vi "Ex4.vi"() -> ()   [LabVIEW 2012]
doc: "Example VI: reads in and writes to Baxter's joint states"
uses:
  <userlib>/ROS for LabVIEW Software/ROS/Code/JointPositions.ctl
  <userlib>/ROS for LabVIEW Software/ROS/Code/Slider.ctl
panel:
  in  "Bring Arms In":bool
  in  "Reset to Zero":bool
  in  "Joint Positions":T1 {"left_w2" scale=-180.0..180.0; "left_w1" scale=-180.0..180.0; "left_w0" scale=-180.0..180.0; "left_e1" scale=-180.0..180.0; "left_e0" scale=-180.0..180.0; "left_s1" scale=-180.0..180.0; "left_s0" scale=-180.0..180.0; "right_s1" scale=-180.0..180.0; "right_s0" scale=-180.0..180.0; "right_w2" scale=-180.0..180.0; "right_e1" scale=-180.0..180.0; "right_e0" scale=-180.0..180.0; "right_w0" scale=-180.0..180.0; "right_w1" scale=-180.0..180.0}
  in  "stop":bool
  # "Control Baxter's Arms using the supplied Position Controller"
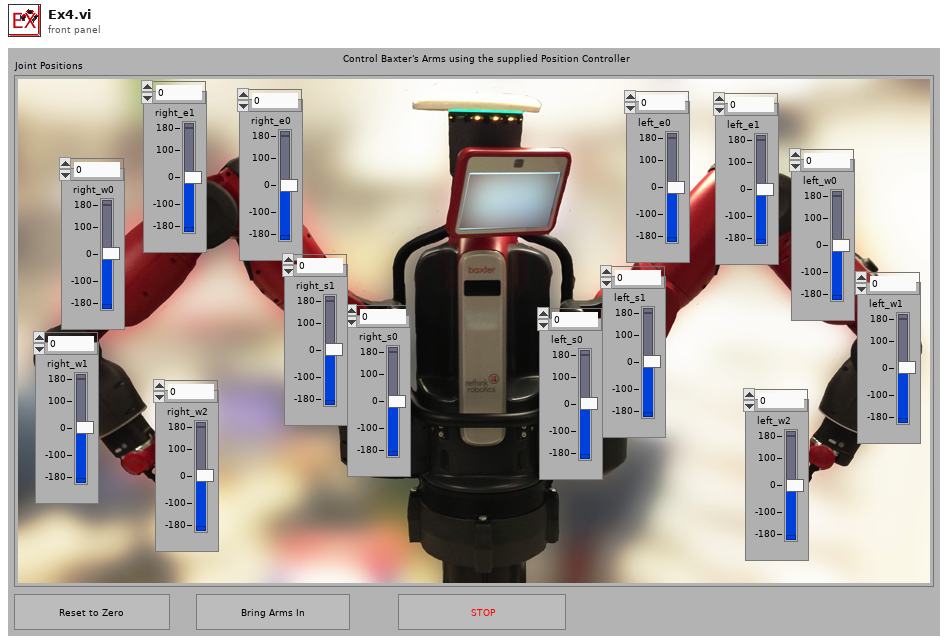
[diagram p1: front panel]
types:
  T1 = typedef "JointPositions.ctl" = cluster{"left_e0":T2, "left_e1":T2, "left_s0":T2, "left_s1":T2, "left_w0":T2, "left_w1":T2, "left_w2":T2, "right_e0":T2, "right_e1":T2, "right_s0":T2, "right_s1":T2, "right_w0":T2, "right_w1":T2, "right_w2":T2}
  T2 = typedef "Slider.ctl" = dbl
  T3 = cluster{"Joint Name":string, "Position":dbl, "Velocity":dbl, "Effort":dbl}[]
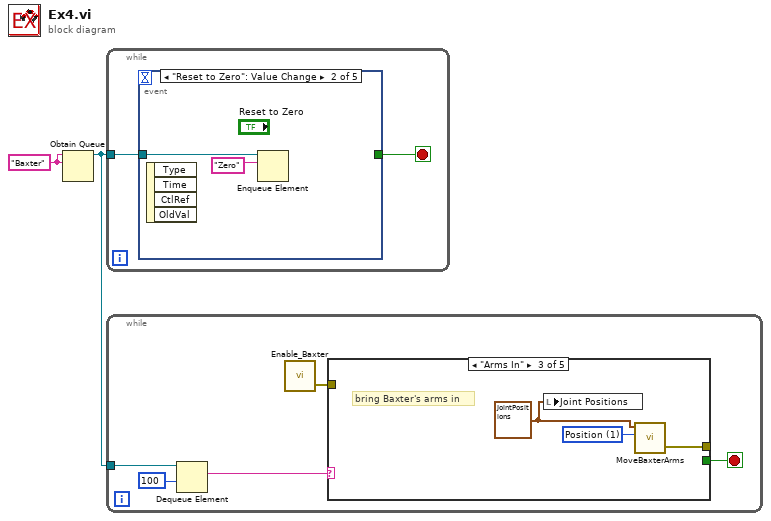
[diagram p0: block diagram]
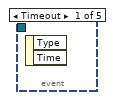
[diagram p2: hidden frame]
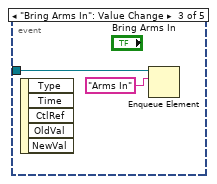
[diagram p3: hidden frame]
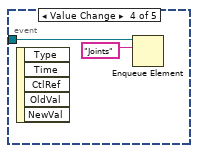
[diagram p4: hidden frame]
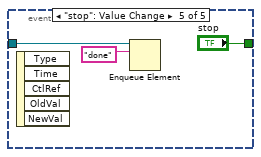
[diagram p5: hidden frame]
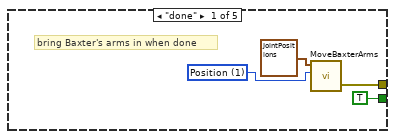
[diagram p6: hidden frame]
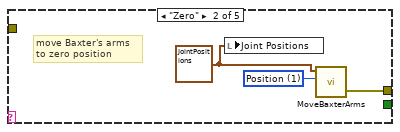
[diagram p7: hidden frame]
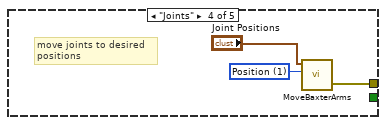
[diagram p8: hidden frame]
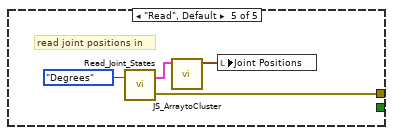
[diagram p9: hidden frame]
diagram:
  w1 = "Baxter" ("name (unnamed)")
  n1 = Obtain Queue(name (unnamed)=w1, element data type=w1) -> (queue out=w2:refnum<queue>)  [unwired: 3 in, 2 out]
  n2 = while {
    tunnel: w2 -> [w3]
    stop <- w4 stop-if-true
    n3 = event shown="[1] \"Reset to Zero\": Value Change" {
      selector: _ -> [_ _ _ _ _]
      dyn-events: _ -> [_ _ _ _ _]
      timeout: _ -> [_ _ _ _ _]
      tunnel: [_ _ _ _ "stop"] -> w4
      tunnel: w3 -> [_ w5 w7 w9 w12]
      event Timeout {
        n4 = event-data() -> ()  [unwired: 1 in, 2 out]
      }
      event "Reset to Zero": Value Change {
        n5 = event-data() -> ()  [unwired: 1 in, 4 out]
        n6 = Enqueue Element(queue=w5, element="Zero") -> ()  [unwired: 2 in, 3 out]
      }
      event "Bring Arms In": Value Change {
        n7 = event-data() -> ()  [unwired: 1 in, 5 out]
        n8 = Enqueue Element(queue=w7, element="Arms In") -> ()  [unwired: 2 in, 3 out]
      }
      event Value Change {
        n9 = event-data() -> ()  [unwired: 1 in, 5 out]
        n10 = Enqueue Element(queue=w9, element="Joints") -> ()  [unwired: 2 in, 3 out]
      }
      event "stop": Value Change {
        n11 = event-data() -> ()  [unwired: 1 in, 5 out]
        n12 = Enqueue Element(queue=w12, element="done") -> ()  [unwired: 2 in, 3 out]
      }
    }
  }
  n13 = while {
    tunnel: w2 -> [w18]
    stop <- w16 stop-if-true
    n14 = Dequeue Element(queue=w18, timeout in ms (-1)=100) -> (element=w17:string)  [unwired: 1 in, 3 out]
    n15 = call <userlib>:"Enable_Baxter.vi"() -> ("error out"=w14:errorcluster)  [unwired: 4 in]
    n16 = case shown="\"Arms In\"" w17 {
      tunnel: [TRUE ("stop") _ _ _ _] -> w16
      tunnel: [w19 w23 w26 w29 w32] -> _
      tunnel: w14 -> [_ _ _ _ _]
      frame "done" {
        w21 = u8 1 items=["Position"=1, "Velocity"=2, "Effort"=3] ("Mode")
        # "bring Baxter's arms in when done"
        n17 = call <userlib>:"MoveBaxterArms.vi"("Parameters"=T1 {"left_e0"=0.0, "left_e1"=90.0, "left_s0"=-30.0, "left_s1"=0.0, "left_w0"=0.0, "left_w1"=0.0, "left_w2"=0.0, "right_e0"=0.0, "right_e1"=90.0, "right_s0"=30.0, "right_s1"=0.0, "right_w0"=0.0, "right_w1"=0.0, "right_w2"=0.0} ("Joint Positions 2"), "Mode"=w21) -> ("error out"=w19:errorcluster)  [unwired: 4 in]
      }
      frame "Zero" {
        w24 = u8 1 items=["Position"=1, "Velocity"=2, "Effort"=3] ("Mode")
        w25 = T1 {"left_e0"=0.0, "left_e1"=0.0, "left_s0"=0.0, "left_s1"=0.0, "left_w0"=0.0, "left_w1"=0.0, "left_w2"=0.0, "right_e0"=0.0, "right_e1"=0.0, "right_s0"=0.0, "right_s1"=0.0, "right_w0"=0.0, "right_w1"=0.0, "right_w2"=0.0} ("Joint Positions 2")
        # "move Baxter's arms\nto zero position"
        n18 = local write "Joint Positions"(w25) -> ()
        n19 = call <userlib>:"MoveBaxterArms.vi"("Parameters"=w25, "Mode"=w24) -> ("error out"=w23:errorcluster)  [unwired: 4 in]
      }
      frame "Arms In" {
        w27 = u8 1 items=["Position"=1, "Velocity"=2, "Effort"=3] ("Mode")
        w28 = T1 {"left_e0"=0.0, "left_e1"=90.0, "left_s0"=-30.0, "left_s1"=0.0, "left_w0"=0.0, "left_w1"=0.0, "left_w2"=0.0, "right_e0"=0.0, "right_e1"=90.0, "right_s0"=30.0, "right_s1"=0.0, "right_w0"=0.0, "right_w1"=0.0, "right_w2"=0.0} ("Joint Positions 2")
        # "bring Baxter's arms in"
        n20 = local write "Joint Positions"(w28) -> ()
        n21 = call <userlib>:"MoveBaxterArms.vi"("Parameters"=w28, "Mode"=w27) -> ("error out"=w26:errorcluster)  [unwired: 4 in]
      }
      frame "Joints" {
        w30 = u8 1 items=["Position"=1, "Velocity"=2, "Effort"=3] ("Mode")
        # "move joints to desired\npositions"
        n22 = call <userlib>:"MoveBaxterArms.vi"("Parameters"="Joint Positions", "Mode"=w30) -> ("error out"=w29:errorcluster)  [unwired: 4 in]
      }
      frame "Read", Default {
        # "read joint positions in"
        n23 = call <userlib>:"Read_Joint_States.vi"("Units (deg)"=enum16{"Radians", "Degrees"}."Degrees") -> ("error out"=w32:errorcluster, "Joint States"=w35:T3)  [unwired: 2 in]
        n24 = call <userlib>:"JS_ArraytoCluster.vi"("Joint States"=w35) -> ("Joint Positions 2"=w33:T1)  [unwired: 10 in]
        n25 = local write "Joint Positions"(w33) -> ()
      }
    }
  }
